vi "Global scale res meter.vi"() -> ()   [LabVIEW 2019]
panel:
  out "FS":T1={"Resistenza1"=2.0, "Resistenza2"=2.0, "RESISTENZA"=2.0}
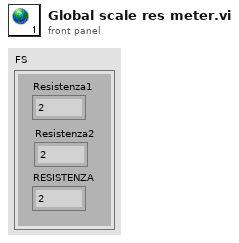
[diagram p1: front panel]
types:
  T1 = cluster{"Resistenza1":dbl, "Resistenza2":dbl, "RESISTENZA":dbl}
diagram:
